vi "Clear all lists.vi"(8 "error in (no error)":errorcluster, 11 "Tamer in":refnum<class "Tamer.lvclass">) -> (0 "error out":errorcluster, 3 "Tamer out":refnum<class "Tamer.lvclass">)   [LabVIEW 2020, in "Tamer.lvlib" / "Tamer.lvclass"]
uses:
  Tamer.lvclass
  Tamer.lvclass/Tamer.ctl
  Run Utilities/TypeDefs/Synchronize FPGA Cluster.ctl
  Run Utilities/Schedule/Schedule.lvclass
  Run Utilities/TypeDefs/Monkey Status.ctl
  Run Utilities/TypeDefs/Messages/Banana Message.ctl
  Run Utilities/TypeDefs/Return Code.ctl
  Run Utilities/TypeDefs/Messages/Script Checker Message.ctl
  Run Utilities/TypeDefs/Script Checker Result.ctl
  Run Utilities/Run Utilities.lvlib
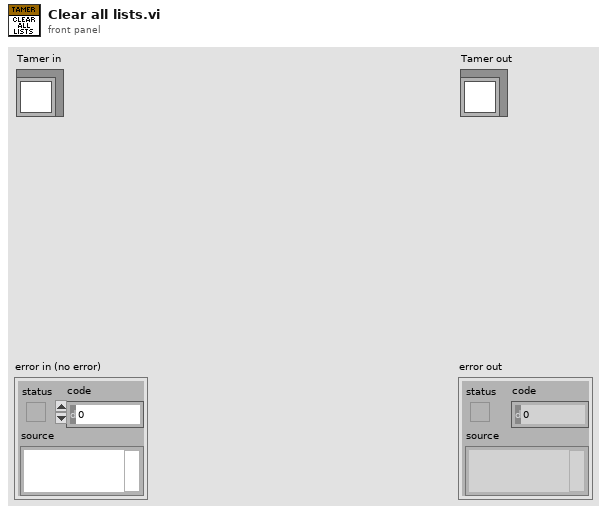
[diagram p1: front panel]
types:
  T1 = typedef "TALOS.lvlib/Run Utilities.lvlib/Script Checker Message.ctl" = cluster{"Monkey ID":string, "Script Checker Result":T2}
  T2 = typedef "TALOS.lvlib/Run Utilities.lvlib/Script Checker Result.ctl" = enum16{"Passed", "Failed", "Empty"}
  T3 = typedef "TALOS.lvlib/Run Utilities.lvlib/Banana Message.ctl" = cluster{"FPGA Name":string, "Return Code":T4}
  T4 = typedef "TALOS.lvlib/Run Utilities.lvlib/Return Code.ctl" = enum16{"All Good", "Retry", "Skip", "Skip All", "ABORT"}
  T5 = typedef "TALOS.lvlib/Run Utilities.lvlib/Monkey Status.ctl" = enum16{"Init", "Paused", "Ongoing", "Stopped", "Finished (no errors)", "Finished (with errors)"}
  T6 = typedef "TALOS.lvlib/Run Utilities.lvlib/Synchronize FPGA Cluster.ctl" = cluster{"Status":bool, "FPGA Name":string}
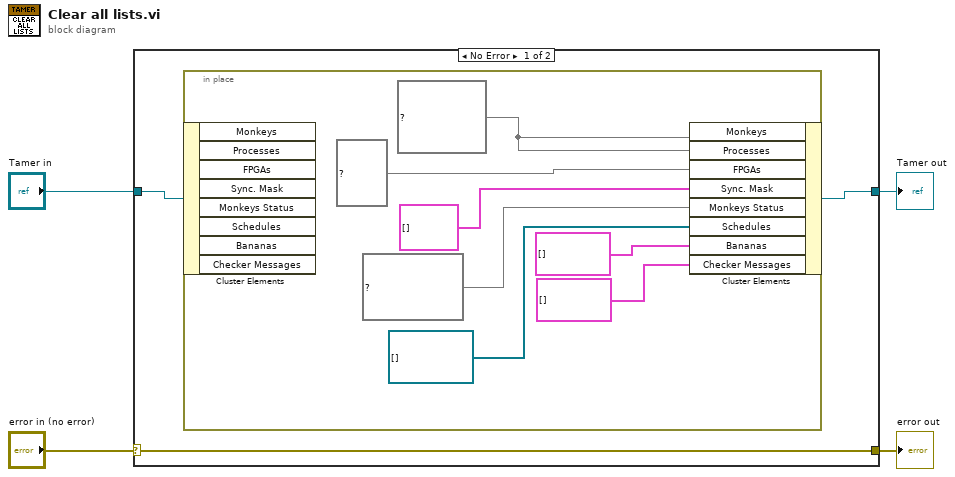
[diagram p0: block diagram]
diagram:
  n1 = case shown="No Error" "error in (no error)" {
    selector: "error in (no error)" -> [w7 w16]
    tunnel: [w7 w16] -> w3
    tunnel: [w5 w15] -> w1
    tunnel: "Tamer in" -> [w6 w15]
    frame No Error {
      n2 = in-place {
        w12 = map{string, string[]} {} ("Monkeys")
        n3 = in-place-cluster #1(w6) -> ()  [unwired: 8 out]
        n4 = in-place-cluster #1("Monkeys"=w12, "Processes"=w12, "FPGAs"=map{string, string} {} ("Kaslis"), "Sync. Mask"=T6[] [], "Monkeys Status"=map{string, T5} {}, "Schedules"=refnum<class "Schedule.lvclass">[] [], "Bananas"=T3[] [], "Checker Messages"=T1[] []) -> (w5:refnum<class "Tamer.lvclass">)
      }
    }
    frame Error {
    }
  }
  "error out" <- w3
  "Tamer out" <- w1
